vi "AnyBuilderBegin.vi"(7 "error in (no error)":errorcluster) -> (0 "error out":errorcluster, 3 "Builder Ref Out":T1)   [LabVIEW 2019, in "TestDataMarshal.lvlib" / "gprc-lvsupport.lvlib"]
uses:
  gprc-lvsupport.lvlib
  typeDefs/grpcId.ctl
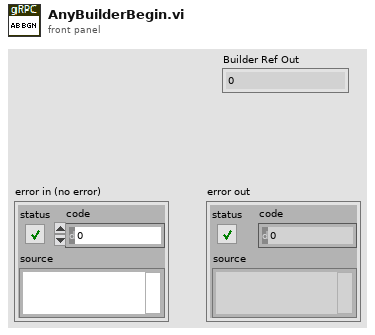
[diagram p1: front panel]
types:
  T1 = typedef "TestDataMarshal.lvlib/gprc-lvsupport.lvlib/grpcId.ctl" = u64
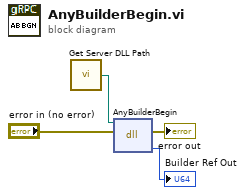
[diagram p0: block diagram]
diagram:
  n1 = call "Get Server DLL Path.vi"() -> ("Server dll path"=w3:path)
  n2 = dll-call lib="?" fn="AnyBuilderBegin"(path in=w3, error in="error in (no error)") -> (error out=→"error out":errorcluster, "anyId"=→"Builder Ref Out":u64)  [unwired: 3 in, 1 out]
